vi "DialogConfigArduino.vi"() -> (0 "Cancel":bool, 1 "Error Out":errorcluster, 2 "Port Name":refnum<visa-resource-name>)   [LabVIEW 2018]
uses:
  <vilib>/Instr/_visa.llb/VISA Configure Serial Port (Instr).vi
panel:
  in  "Cancel Button":bool
  in  "Save Button":bool
  in  "Baud rate":dbl
  in  "COM Port":refnum<visa-resource-name>
  # "CONEXÃO COM O ARDUINO"
  # "PORTA"
  # "BAUD RATE"
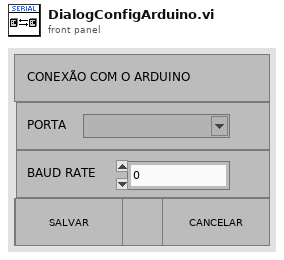
[diagram p1: front panel]
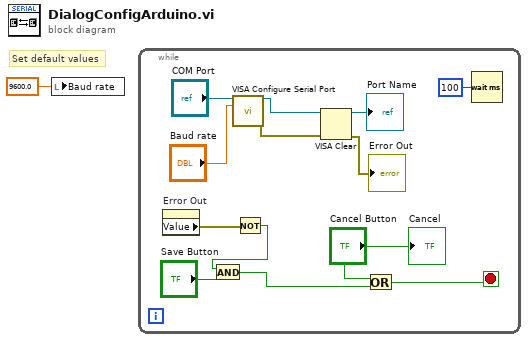
[diagram p0: block diagram]
diagram:
  # "Set default values"
  n1 = local write "Baud rate"(9600.0 ("Baud rate")) -> ()
  n2 = while {
    stop <- w4 stop-if-true
    n3 = property on="Error Out" class="Clust (strict)"() -> ("Value"=w6:errorcluster)  [unwired: 2 in, 2 out]
    n4 = call-poly "VISA Configure Serial Port"("VISA resource name"="COM Port", "baud rate (9600)"="Baud rate") -> ("VISA resource name out"=w12:refnum<visa-resource-name>, "error out"=w9:errorcluster)  [unwired: 12 in]
    n5 = Not(x=w6) -> (.not. x?=w5:bool)
    n6 = And(x=w5, y="Save Button") -> (x .and. y?=w3:bool)
    n7 = VISA Clear(VISA resource name=w12, error in (no error)=w9) -> (VISA resource name out=→"Port Name":refnum<visa-resource-name>, error out=→"Error Out":errorcluster)
    n8 = Or(x="Cancel Button", y=w3) -> (x .or. y?=w4:bool)
    n9 = Wait (ms)(milliseconds to wait=u32 100) -> ()  [unwired: 1 out]
    "Cancel" <- "Cancel Button"
  }
